vi "Main.vi"() -> ()   [LabVIEW 2014]
uses:
  Control numerico.ctl
  Indicador numerico.ctl
  Controle sinal.ctl
  <vilib>/Analysis/polynomials.llb/Polynomial Plot (Range).vi
  <vilib>/Analysis/polynomials.llb/Polynomial Roots (DBL).vi
  <vilib>/Analysis/NI_AALPro.lvlib
panel:
  in  "Sinal a2":T1="+"
  in  "Sinal a0":T1="+"
  in  "Sinal a1":T1="+"
  in  "a2":T2=1.0 min=-1.0 max=999.0
  in  "a1":T2=10.0 min=-1.0 max=999.0
  in  "a0":T2=25.0 min=-1.0 max=999.0
  out "x1":T3 format="%#_3g"
  out "x2":T3 format="%#_3g"
  out "XY Graph":cluster{"Ramp Pattern":dbl[], "P(A)":dbl[]}[](graph)
  # "Equação de segundo grau"
  # "Raizes:"
  # "x1  ="
  # "x2  ="
  # "0"
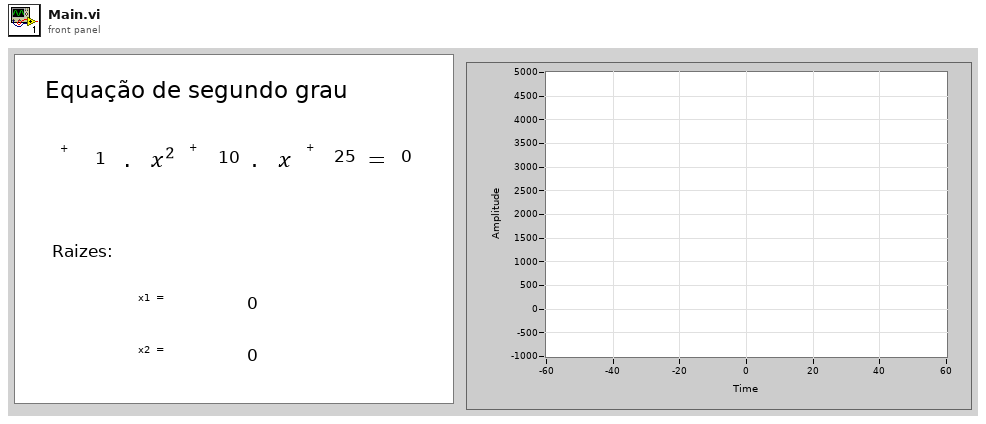
[diagram p1: front panel]
types:
  T1 = typedef "Controle sinal.ctl" = string
  T2 = typedef "Control numerico.ctl" = dbl
  T3 = typedef "Indicador numerico.ctl" = cdb
  T4 = cluster{"cmd":string, "a0":dbl, "a1":dbl, "a2":dbl, "Sinal a0":i32, "Sinal a1":i32, "Sinal a2":i32}
  T5 = enum8{"Enabled", "Disabled", "Disabled and Grayed Out"}
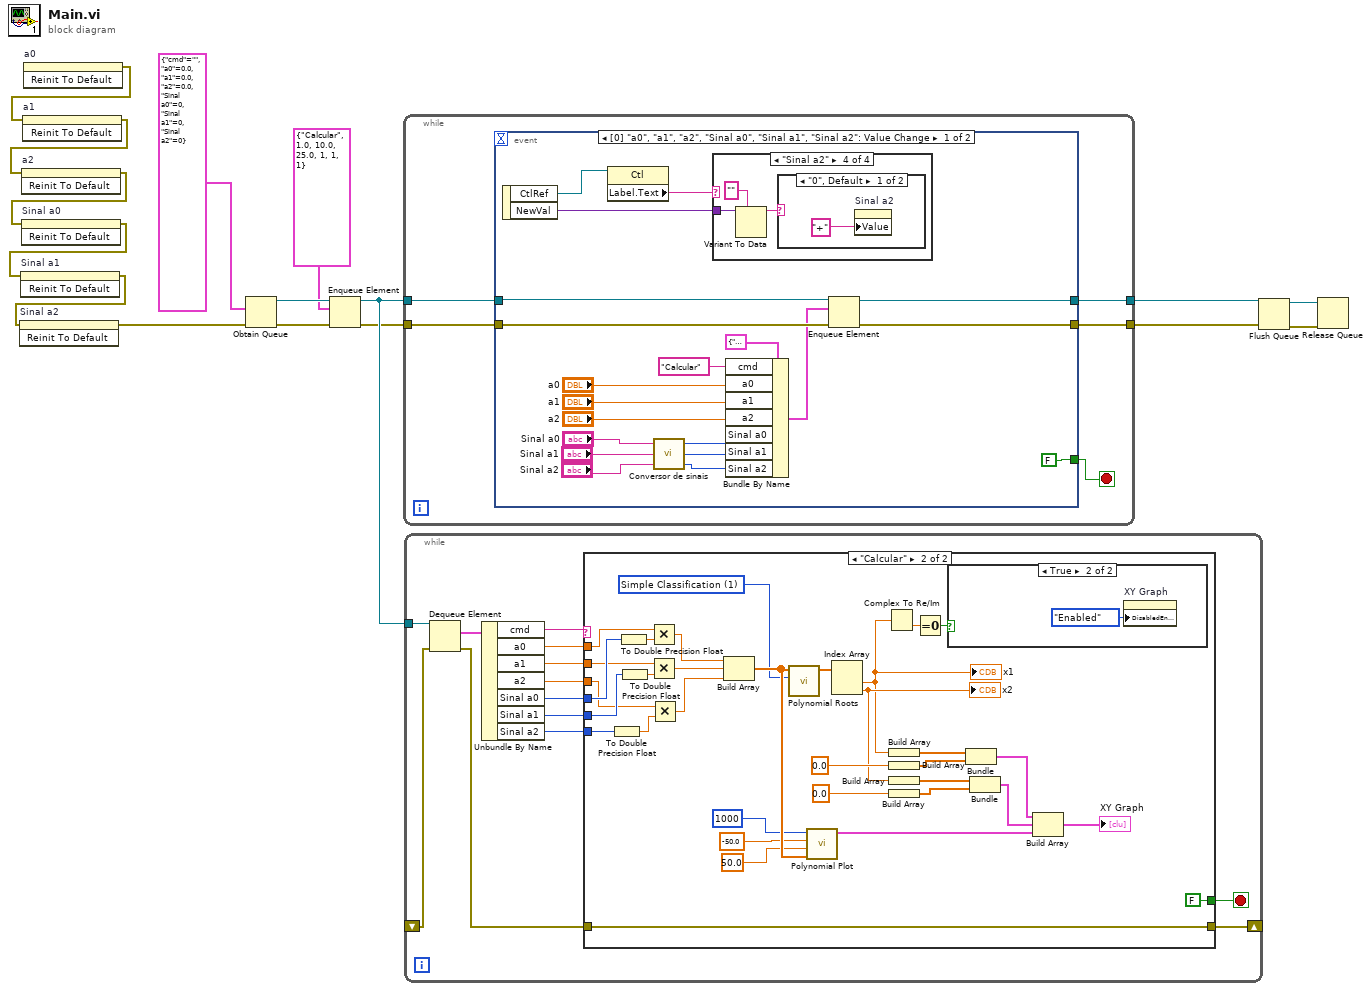
[diagram p0: block diagram]
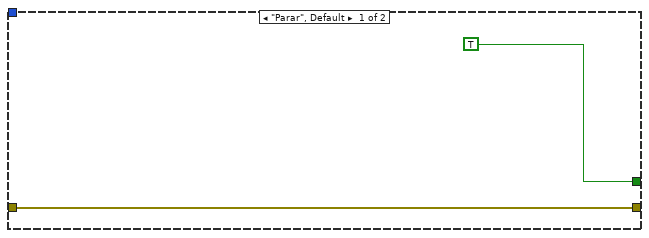
[diagram p2: hidden frame]
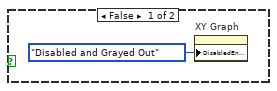
[diagram p3: hidden frame]
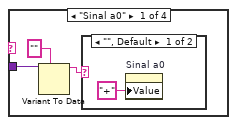
[diagram p4: hidden frame]
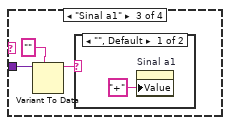
[diagram p7: hidden frame]
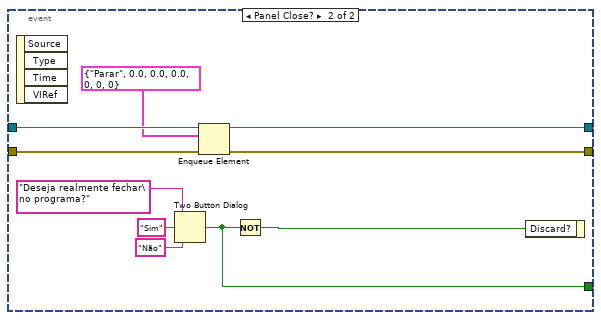
[diagram p10: hidden frame]
diagram:
  n1 = invoke on="a0" class="DigNum (strict)" method="Reinit To Default"() -> (error out=w7:errorcluster)  [unwired: 3 in, 2 out]
  n2 = invoke on="a1" class="DigNum (strict)" method="Reinit To Default"(error in=w7) -> (error out=w6:errorcluster)  [unwired: 2 in, 2 out]
  n3 = invoke on="a2" class="DigNum (strict)" method="Reinit To Default"(error in=w6) -> (error out=w5:errorcluster)  [unwired: 2 in, 2 out]
  n4 = invoke on="Sinal a0" class="Str (strict)" method="Reinit To Default"(error in=w5) -> (error out=w4:errorcluster)  [unwired: 2 in, 2 out]
  n5 = invoke on="Sinal a1" class="Str (strict)" method="Reinit To Default"(error in=w4) -> (error out=w2:errorcluster)  [unwired: 2 in, 2 out]
  n6 = invoke on="Sinal a2" class="Str (strict)" method="Reinit To Default"(error in=w2) -> (error out=w1:errorcluster)  [unwired: 2 in, 2 out]
  n7 = Obtain Queue(element data type=T4 {"cmd"="", "a0"=0.0, "a1"=0.0, "a2"=0.0, "Sinal a0"=0, "Sinal a1"=0, "Sinal a2"=0}, error in (no error)=w1) -> (queue out=w11:refnum<queue>, error out=w12:errorcluster)  [unwired: 3 in, 1 out]
  n8 = Enqueue Element(queue=w11, element=T4 {"cmd"="Calcular", "a0"=1.0, "a1"=10.0, "a2"=25.0, "Sinal a0"=1, "Sinal a1"=1, "Sinal a2"=1}, error in (no error)=w12) -> (queue out=w10:refnum<queue>, error out=w9:errorcluster)  [unwired: 1 in, 1 out]
  n9 = while {
    tunnel: w10 -> [w20]
    tunnel: w9 -> [w21]
    tunnel: [w19] -> w16
    tunnel: [w18] -> w15
    stop <- w17 stop-if-true
    n10 = event shown="[0] \"a0\", \"a1\", \"a2\", \"Sinal a0\", \"Sinal a1\", \"Sinal a2\": Value Change" {
      selector: _ -> [_ _]
      dyn-events: _ -> [_ _]
      timeout: _ -> [_ _]
      tunnel: w21 -> [w37 w55]
      tunnel: w20 -> [w38 w56]
      tunnel: [w41 w58] -> w19
      tunnel: [w40 w57] -> w18
      tunnel: [FALSE ("stop") w59] -> w17
      event Value Change {
        n11 = event-data() -> ("CtlRef"=w33:refnum<vi>, "NewVal"=w32:variant)  [unwired: 1 in]
        n12 = property class="Ctl"(reference=w33) -> ("Label.Text"=w34:string)  [unwired: 1 in, 2 out]
        n13 = call "Conversor de sinais.vi"("Sinal a2"="Sinal a2", "Sinal a1"="Sinal a1", "Sinal a0"="Sinal a0") -> ("Sinal a2"=w22:i32, "Sinal a1"=w27:i32, "Sinal a0"=w28:i32)
        n14 = case shown="\"Sinal a2\"" w34 {
          tunnel: w32 -> [w43 _ w48 w50]
          frame "Sinal a0" {
            n15 = Variant To Data(type="", Variant=w43) -> (data=w42:string)  [unwired: 1 in, 1 out]
            n16 = case shown="\"\", Default" w42 {
              frame "", Default {
                n17 = property on="Sinal a0" class="Str (strict)"("Value"=T1 "+" ("Sinal a0")) -> ()  [unwired: 2 in, 2 out]
              }
              frame "+", "-" {
              }
            }
          }
          frame "0", Default {
          }
          frame "Sinal a1" {
            n18 = Variant To Data(type="", Variant=w48) -> (data=w46:string)  [unwired: 1 in, 1 out]
            n19 = case shown="\"\", Default" w46 {
              frame "", Default {
                n20 = property on="Sinal a1" class="Str (strict)"("Value"=T1 "+" ("Sinal a1")) -> ()  [unwired: 2 in, 2 out]
              }
              frame "+", "-" {
              }
            }
          }
          frame "Sinal a2" {
            n21 = Variant To Data(type="", Variant=w50) -> (data=w51:string)  [unwired: 1 in, 1 out]
            n22 = case shown="\"0\", Default" w51 {
              frame "0", Default {
                n23 = property on="Sinal a2" class="Str (strict)"("Value"=T1 "+" ("Sinal a1")) -> ()  [unwired: 2 in, 2 out]
              }
              frame "+", "-" {
              }
            }
          }
        }
        n24 = Bundle By Name(cluster=T4 {"cmd"="Calcular", "a0"=1.0, "a1"=10.0, "a2"=25.0, "Sinal a0"=1, "Sinal a1"=1, "Sinal a2"=1} ("element"), "cmd"="Calcular", "a0"="a0", "a1"="a1", "a2"="a2", "Sinal a0"=w28, "Sinal a1"=w27, "Sinal a2"=w22) -> (w35:T4)
        n25 = Enqueue Element(queue=w38, element=w35, error in (no error)=w37) -> (queue out=w41:refnum<queue>, error out=w40:errorcluster)  [unwired: 1 in, 1 out]
      }
      event Panel Close? {
        n26 = event-data() -> ()  [unwired: 1 in, 4 out]
        n27 = Two Button Dialog(message="Deseja realmente fechar\no programa?", 1:"Não" ("F button name (\"Cancel\")"), 2:"Sim" ("T button name (\"OK\")")) -> (T button?=w59:bool)
        n28 = Enqueue Element(queue=w56, element=T4 {"cmd"="Parar", "a0"=0.0, "a1"=0.0, "a2"=0.0, "Sinal a0"=0, "Sinal a1"=0, "Sinal a2"=0}, error in (no error)=w55) -> (queue out=w58:refnum<queue>, error out=w57:errorcluster)  [unwired: 1 in, 1 out]
        n29 = Not(x=w59) -> (.not. x?=w60:bool)
        n30 = event-data("Discard?"=w60) -> ()  [unwired: 1 in, 1 out]
      }
    }
  }
  n31 = while {
    tunnel: w10 -> [w76]
    shift-right: [w73] -> _
    shift-left: _ -> [w75]
    stop <- w72 stop-if-true
    n32 = Dequeue Element(queue=w76, error in (no error)=w75) -> (element=w71:T4, error out=w74:errorcluster)  [unwired: 1 in, 2 out]
    n33 = Unbundle By Name(w71) -> ("cmd"=w70:string, "a0"=w69:dbl, "a1"=w68:dbl, "a2"=w67:dbl, "Sinal a0"=w66:i32, "Sinal a1"=w65:i32, "Sinal a2"=w64:i32)
    n34 = case shown="\"Calcular\"" w70 {
      tunnel: w74 -> [w78 w111]
      tunnel: [w78 w111] -> w73
      tunnel: [TRUE FALSE] -> w72
      tunnel: w69 -> [_ w109]
      tunnel: w68 -> [_ w107]
      tunnel: w67 -> [_ w80]
      tunnel: w66 -> [_ w110]
      tunnel: w65 -> [_ w106]
      tunnel: w64 -> [_ w81]
      frame "Parar", Default {
      }
      frame "Calcular" {
        w83 = u16 1 items=["General", "Simple Classification", "Refinement", "Advanced Refinement"] ("option")
        n35 = To Double Precision Float(number=w81) -> (double precision float=w82:dbl)
        n36 = To Double Precision Float(number=w110) -> (double precision float=w108:dbl)
        n37 = To Double Precision Float(number=w106) -> (double precision float=w105:dbl)
        n38 = Multiply(x=w109, y=w108) -> (x*y=w104:dbl)
        n39 = Multiply(x=w107, y=w105) -> (x*y=w103:dbl)
        n40 = Multiply(x=w80, y=w82) -> (x*y=w79:dbl)
        n41 = Build Array(w104, w103, w79) -> (w101:dbl[])
        n42 = call-poly <vilib>:"Polynomial Roots.vi"("option"=w83, "P(x)"=w101) -> ("Roots"=w102:cdb[])  [unwired: 8 in, 1 out]
        n43 = call-poly <vilib>:"Polynomial Plot.vi"("P(x)"=w101, "end"=50.0, "start"=-50.0, "samples"=1000) -> ("polynomial plot"=w97:cluster{"Ramp Pattern":dbl[], "P(A)":dbl[]})  [unwired: 6 in, 1 out]
        n44 = Index Array(array=w102) -> (element #1=w86:cdb, element #2=w87:cdb)  [unwired: 2 in]
        "x2" <- w87
        "x1" <- w86
        n45 = Complex To Re/Im(x + iy=w86) -> (y=w85:dbl)  [unwired: 1 out]
        n46 = Build Array(w86) -> (w90:cdb[])
        n47 = Build Array(0.0 ("element")) -> (w91:dbl[])
        n48 = Build Array(w87) -> (w95:cdb[])
        n49 = Build Array(0.0 ("element")) -> (w94:dbl[])
        n50 = Equal To 0?(x=w85) -> (x = 0?=w84:bool)
        n51 = case shown="True" w84 {
          frame False {
            n52 = property on="XY Graph" class="XYGraph (strict)"("DisabledEnum"=T5."Disabled and Grayed Out" ("Disabled")) -> ()  [unwired: 2 in, 2 out]
          }
          frame True {
            n53 = property on="XY Graph" class="XYGraph (strict)"("DisabledEnum"=T5."Enabled" ("Disabled")) -> ()  [unwired: 2 in, 2 out]
          }
        }
        n54 = Bundle(w90, w91) -> (w88:cluster{cdb[], dbl[]})  [unwired: 1 in]
        n55 = Bundle(w95, w94) -> (w93:cluster{cdb[], dbl[]})  [unwired: 1 in]
        n56 = Build Array(w88, w93, w97) -> (→"XY Graph":cluster{"Ramp Pattern":cdb[], "P(A)":dbl[]}[])
      }
    }
  }
  n57 = Flush Queue(queue=w16, error in (no error)=w15) -> (queue out=w14:refnum<queue>, error out=w13:errorcluster)  [unwired: 1 out]
  n58 = Release Queue(queue=w14, error in (no error)=w13) -> ()  [unwired: 1 in, 3 out]
